vi "Valid Measurement Service Name.vi"(8 "error in":errorcluster, 10 "requested plugin name":string, 11 "project ref":refnum<vi>) -> (0 "error out":errorcluster, 3 "valid name?":bool)   [LabVIEW 2021, in "G-Plugin Editor.lvlib"]
uses:
  G-Plugin Editor.lvlib
  48953c88-0603-4c13-ba6a-df914321b09e.vi
  <vilib>/Comparison/Equal/Equal Functor/Equal Functor.lvclass
panel:
  out "control chars":string
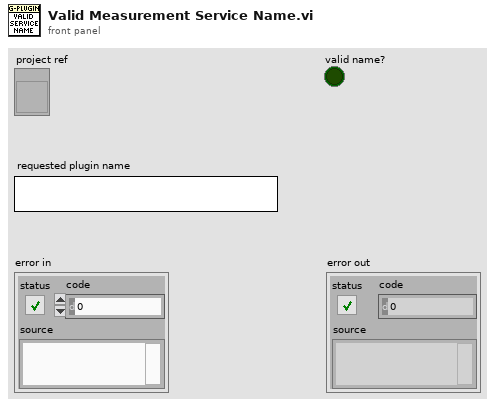
[diagram p1: front panel]
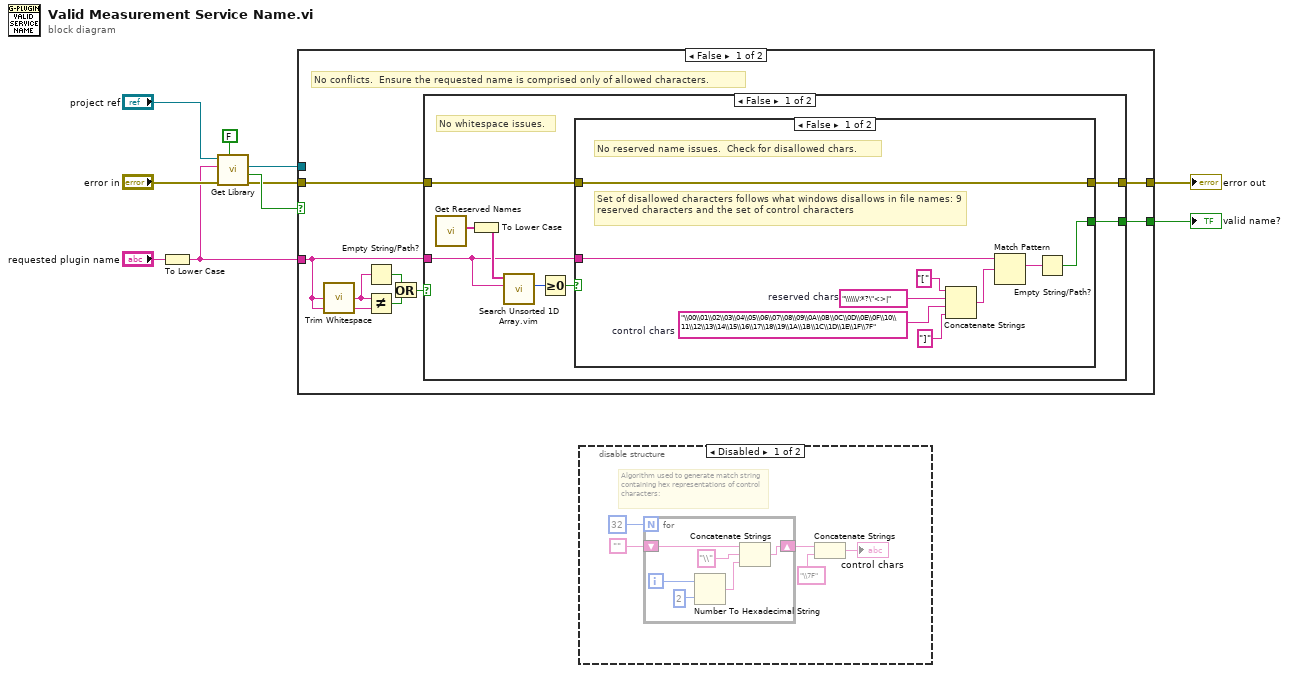
[diagram p0: block diagram]
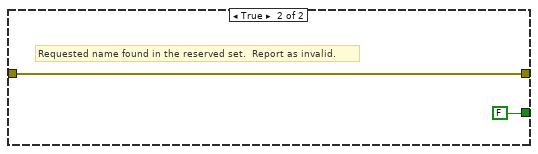
[diagram p3: hidden frame]
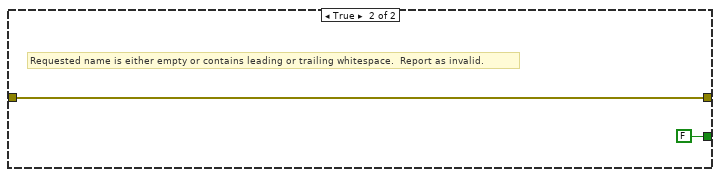
[diagram p4: hidden frame]
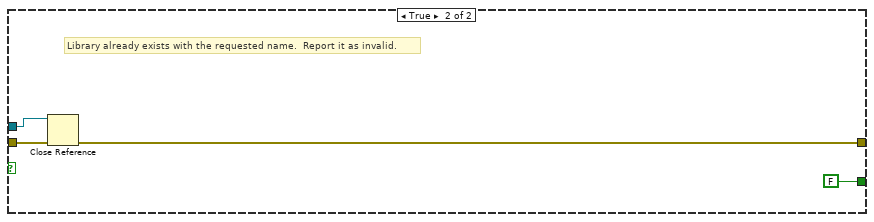
[diagram p5: hidden frame]
diagram:
  n1 = To Lower Case(string="requested plugin name") -> (all lower case string=w1:string)
  n2 = call "Get Library.vi"("error if not found"=FALSE ("Error if not Found (T)"), "error in (no error)"="error in", "library name"=w1, "project ref"="project ref") -> ("error out"=w7:errorcluster, "found"=w8:bool, "library item"=w6:refnum<vi>)  [unwired: 4 in, 1 out]
  n3 = case shown="False" w8 {
    tunnel: w7 -> [w18 w43]
    tunnel: w6 -> [_ w41]
    tunnel: [w17 w42] -> w4
    tunnel: [w16 FALSE ("Valid Name?")] -> w3
    tunnel: w1 -> [w11 _]
    frame False {
      # "No conflicts.  Ensure the requested name is comprised only of allowed characters."
      n4 = call <vilib>:"Trim Whitespace.vi"("string"=w11) -> ("trimmed string"=w15:string)  [unwired: 1 in]
      n5 = Empty String/Path?(string/path=w15) -> (empty?=w13:bool)
      n6 = Not Equal?(x=w15, y=w11) -> (x != y?=w14:bool)
      n7 = Or(x=w13, y=w14) -> (x .or. y?=w12:bool)
      n8 = case shown="False" w12 {
        tunnel: w11 -> [w22 _]
        tunnel: w18 -> [w26 w39]
        tunnel: [w25 w39] -> w17
        tunnel: [w19 FALSE ("Error if not Found (T)")] -> w16
        frame False {
          # "No whitespace issues."
          n9 = call "Get Reserved Names.vi"() -> ("reserved names"=w24:string[])  [unwired: 11 in]
          n10 = To Lower Case(string=w24) -> (all lower case string=w23:string[])
          n11 = call "Search Unsorted 1D Array.vim"("element"=w22, "unsorted 1D array"=w23) -> ("index of element"=w21:i32)  [unwired: 9 in]
          n12 = Greater Or Equal To 0?(x=w21) -> (x >= 0?=w20:bool)
          n13 = case shown="False" w20 {
            tunnel: w22 -> [w34 _]
            tunnel: w26 -> [w35 w37]
            tunnel: [w35 w37] -> w25
            tunnel: [w32 FALSE ("Error if not Found (T)")] -> w19
            frame False {
              w27 = "\\00\\01\\02\\03\\04\\05\\06\\07\\08\\09\\0A\\0B\\0C\\0D\\0E\\0F\\10\\11\\12\\13\\14\\15\\16\\17\\18\\19\\1A\\1B\\1C\\1D\\1E\\1F\\7F"  # control chars
              w31 = "\\\\\\/:*?\"<>|"  # reserved chars
              # "Set of disallowed characters follows what windows disallows in file names: 9 reserved characters and the set of control characters"
              # "No reserved name issues.  Check for disallowed chars."
              n14 = Concatenate Strings("[" ("string"), w31, w27, "]" ("string")) -> (w28:string)
              n15 = Match Pattern(string=w34, regular expression=w28) -> (match substring=w33:string)  [unwired: 1 in, 3 out]
              n16 = Empty String/Path?(string/path=w33) -> (empty?=w32:bool)
            }
            frame True {
              # "Requested name found in the reserved set.  Report as invalid."
            }
          }
        }
        frame True {
          # "Requested name is either empty or contains leading or trailing whitespace.  Report as invalid."
        }
      }
    }
    frame True {
      # "Library already exists with the requested name.  Report it as invalid."
      n17 = Close Reference(reference=w41, error in (no error)=w43) -> (error out=w42:errorcluster)
    }
  }
  "error out" <- w4
  "valid name?" <- w3
  n18 = disable-structure shown="Disabled" {
    frame Disabled {
      # "Algorithm used to generate match string containing hex representations of control characters:"
      n19 = for {
        N: 32 -> [_]
        shift-right: [w50] -> w46
        shift-left: "" -> [w49]
        i -> [w54]
        n20 = Number To Hexadecimal String(1:i16 2 ("width (-)"), 2:w54) -> (0:w52:string)
        n21 = Concatenate Strings(w49, "\\" ("string"), w52) -> (w50:string)
      }
      n22 = Concatenate Strings(w46, "\\7F") -> (→"control chars":string)
    }
    frame Enabled {
    }
  }
